vi "cluster in place.vi"   [LabVIEW 2013]
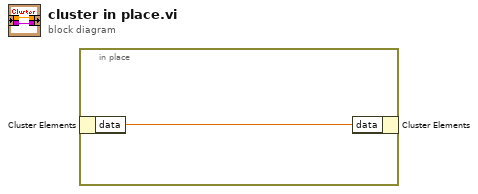
[diagram p0: block diagram]
diagram:
  n1 = in-place {
    n2 = in-place-cluster #1() -> ("data"=w1:dbl)  [unwired: 1 in]
    n3 = in-place-cluster #1("data"=w1) -> ()  [unwired: 1 out]
  }
